vi "例7-2.vi"() -> ()   [LabVIEW 2019]
uses:
  <vilib>/Instr/_visa.llb/VISA Configure Serial Port (Instr).vi
panel:
  in  "VISA resource name":refnum<visa-resource-name> caption="VISA资源名称"
  in  "停止":bool
  in  "发送":bool
  out "接收信息区":string
  in  "发送信息区":string="收到信息请回复--收到信息"
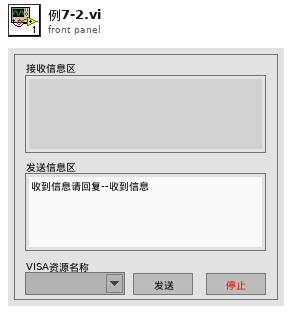
[diagram p1: front panel]
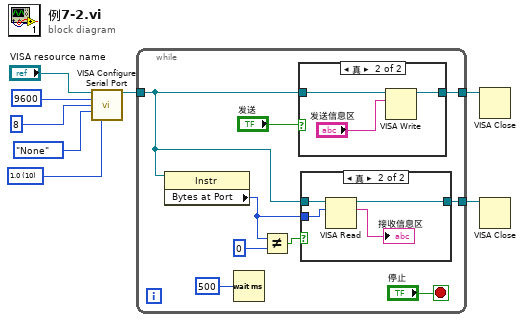
[diagram p0: block diagram]
diagram:
  w5 = u16 10 items=["1.0"=10, "1.5"=15, "2.0"=20] ("stop bits (10: 1 bit)")
  n1 = call-poly "VISA Configure Serial Port"("VISA resource name"="VISA resource name", "baud rate (9600)"=u32 9600, "data bits (8)"=u16 8, "parity (0:none)"=enum16{"None", "Odd", "Even", "Mark", "Space"}."None", "stop bits (10: 1 bit)"=w5) -> ("VISA resource name out"=w8:refnum<visa-resource-name>)  [unwired: 9 in, 1 out]
  n2 = while {
    tunnel: w8 -> [w10]
    tunnel: [w14] -> w7
    tunnel: [w11] -> w6
    stop <- "停止" stop-if-true
    n3 = property class="Instr"(reference=w10) -> ("Bytes at Port"=w9:u32)  [unwired: 1 in, 2 out]
    n4 = Wait (ms)(milliseconds to wait=500) -> ()  [unwired: 1 out]
    n5 = Not Equal?(x=w9, y=0) -> (x != y?=w13:bool)
    n6 = case shown="真" "发送" {
      tunnel: w10 -> [w23 w26]
      tunnel: [w23 w24] -> w14
      frame False {
      }
      frame True {
        n7 = VISA Write(VISA resource name=w26, write buffer="发送信息区") -> (VISA resource name out=w24:refnum<visa-resource-name>)  [unwired: 1 in, 2 out]
      }
    }
    n8 = case shown="真" w13 {
      tunnel: w10 -> [w18 w22]
      tunnel: [w18 w20] -> w11
      tunnel: w9 -> [_ w19]
      frame False {
      }
      frame True {
        n9 = VISA Read(VISA resource name=w22, byte count=w19) -> (VISA resource name out=w20:refnum<visa-resource-name>, read buffer=→"接收信息区":string)  [unwired: 1 in, 2 out]
      }
    }
  }
  n10 = VISA Close(VISA resource name=w7) -> ()  [unwired: 1 in, 1 out]
  n11 = VISA Close(VISA resource name=w6) -> ()  [unwired: 1 in, 1 out]
